vi "ShowRecord.vi"(0 "reference in":refnum<class "CustomersData.lvclass">, 5 "error in (no error)":errorcluster) -> (14 "reference out":refnum<class "CustomersData.lvclass">, 19 "error out":errorcluster)   [LabVIEW 2020, in "CustomersData.lvclass"]
uses:
  CustomersData.lvclass
  C:/Projects/DesignPatterns_Trunk/Bridge/DataObject_class/DataObject.lvclass
  DataObject_class/DataObject.lvclass
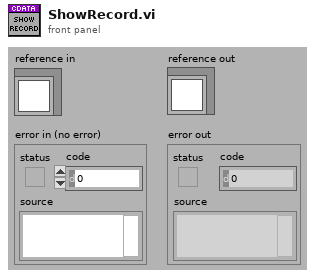
[diagram p1: front panel]
types:
  T1 = typedef "CustomersData.lvclass/ObjectAttributes.ctl" = cluster{"_customers":string[], "_current":i32}
  T2 = typedef "DataObject.lvclass/ObjectAttributes.ctl" = cluster{"StringRef":refnum<vi>}
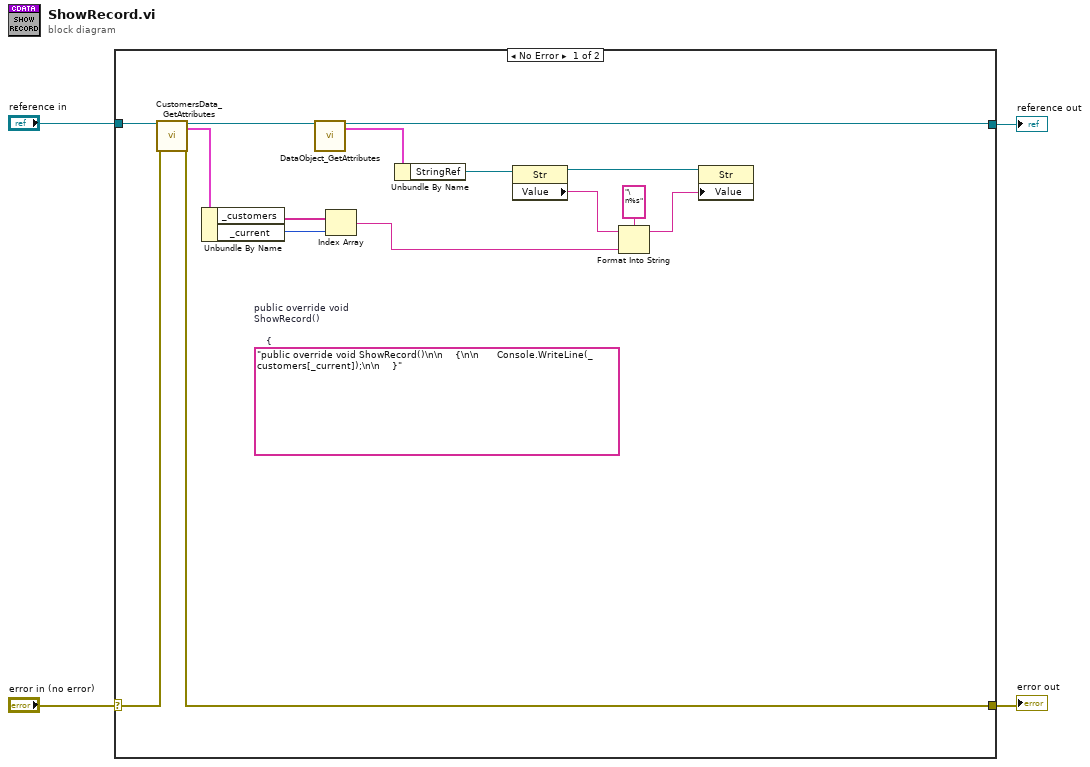
[diagram p0: block diagram]
diagram:
  n1 = case shown="No Error" "error in (no error)" {
    selector: "error in (no error)" -> [w18 w21]
    tunnel: [w15 w21] -> w3
    tunnel: [w12 w20] -> w1
    tunnel: "reference in" -> [w19 w20]
    frame No Error {
      (unwired) "public override void ShowRecord()\n\n    {\n\n      Console.WriteLine(_customers[_current]);\n\n    }"  # public override void ShowRecord()      {        Console.WriteLine(_customers[_current]);      }
      n2 = call "CustomersData_GetAttributes.vi"("reference in"=w19, "error in (no error)"=w18) -> ("reference out"=w16:refnum<class "CustomersData.lvclass">, "Data"=w17:T1, "error out"=w15:errorcluster)  [unwired: 14 in, 1 out]
      n3 = Unbundle By Name(w17) -> ("_customers"=w14:string[], "_current"=w13:i32)
      n4 = call "DataObject_GetAttributes.vi"("reference in"=w16) -> ("reference out"=w12:refnum<class "CustomersData.lvclass">, "Data"=w11:T2)  [unwired: 15 in, 2 out]
      n5 = Index Array(array=w14, index=w13) -> (element=w8:string)
      n6 = Unbundle By Name(w11) -> ("StringRef"=w10:refnum<vi>)
      n7 = property class="Str"(reference=w10) -> (reference out=w9:refnum<vi>, "Value"=w7:string)  [unwired: 1 in, 1 out]
      n8 = Format Into String(format string="\n%s", initial string=w7, w8) -> (resulting string=w6:string)  [unwired: 1 in, 1 out]
      n9 = property class="Str"(reference=w9, "Value"=w6) -> ()  [unwired: 1 in, 2 out]
    }
    frame Error {
    }
  }
  "error out" <- w3
  "reference out" <- w1
